vi "Waveform, Filter Moving Average.vi"(5 "Average Size":dbl=10.0, 6 "error in":errorcluster, 9 "waveform":waveform(dbl)={"t0"=timestamp(3472747248.0780005 s since 1904-01-01), "dt"=2e-06, "Y"=[]}) -> (0 "error out":errorcluster, 3 "waveform out":waveform(dbl)={"t0"=timestamp(0 s since 1904-01-01), "dt"=1.0, "Y"=[]})   [LabVIEW 2010]
doc: "This function filters a waveform using a moving average (implemented with the LabVIEW FIR Filter function)."
uses:
  <vilib>/Analysis/3filter.llb/FIR Filter (DBL).vi
  <vilib>/Analysis/NI_AALBase.lvlib
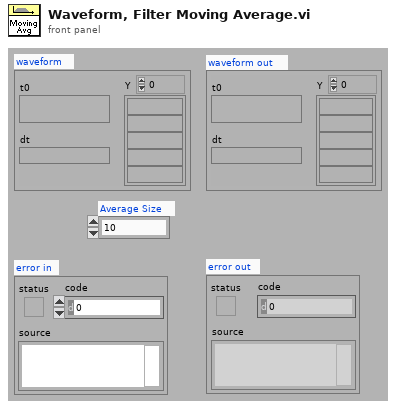
[diagram p1: front panel]
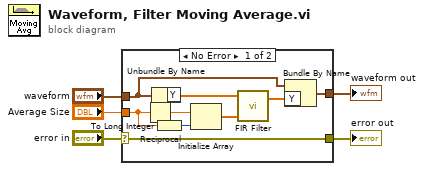
[diagram p0: block diagram]
diagram:
  n1 = case shown="No Error" "error in" {
    selector: "error in" -> [w6 w15]
    tunnel: [w12 _] -> w5
    tunnel: "waveform" -> [w9 _]
    tunnel: "Average Size" -> [w8 _]
    tunnel: [w6 w15] -> w1
    frame No Error {
      n2 = Reciprocal(x=w8) -> (1/x=w14:dbl)
      n3 = Unbundle By Name(w9) -> ("Y"=w10:dbl[])
      n4 = To Long Integer(number=w8) -> (32bit integer=w7:i32)
      n5 = Initialize Array(w14, w7) -> (w13:dbl[])
      n6 = call-poly <vilib>:"FIR Filter.vi"("FIR Coefficients"=w13, "X"=w10) -> ("Filtered X"=w11:dbl[])  [unwired: 2 in, 1 out]
      n7 = Bundle By Name(cluster=w9, "Y"=w11) -> (w12:waveform(dbl))
    }
    frame Error {
    }
  }
  "waveform out" <- w5
  "error out" <- w1
